vi "create Legend.vi"(8 "error in (no error)":errorcluster, 11 "Chart Options":T1={"ChartName"="Chart", "BorderDashStyle"=enum."Solid", "Bordercolor"=0, "Title"={"Title"="", "TitleFontSize"=0.0, "fontName"="Arial", "font Color"=0, "Docking"=enum."Top"}, "Legend"={"Docking"=enum."None", "BorderDashStyle"=enum."Solid", "BGKcolor"=0, "BGKalpha"=103, "Title"="", "TitleSeparator"=enum."ThickLine"}} {"Legend"."BGKalpha" scale=0.0..255.0; "Title"."TitleFontSize" min=4.0 max=100.0}) -> (0 "error out":errorcluster, 3 ".NET MSChart Legend":refnum<k24>)   [LabVIEW 2015, in "Graph Extensions MSChart.lvlib"]
uses:
  Graph Extensions MSChart.lvlib
  System.Windows.Forms.DataVisualization
  Controls/Chart.ctl
  Controls/Title.ctl
  Controls/Legend.ctl
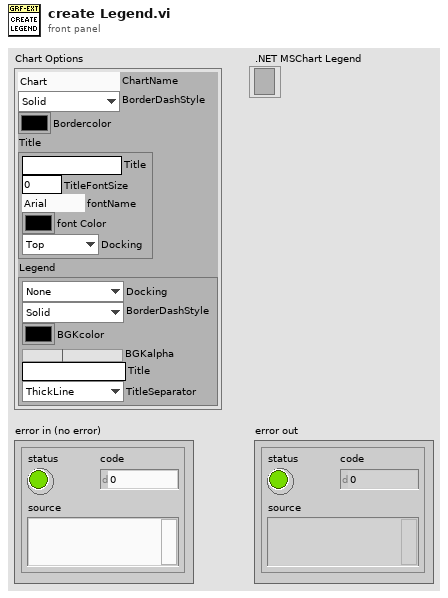
[diagram p1: front panel]
types:
  T1 = typedef "Graph Extensions MSChart.lvlib/Chart.ctl" = cluster{"ChartName":string, "BorderDashStyle":enum16{"NotSet", "Dash", "DashDot", "DashDotDot", "Dot", "Solid"}, "Bordercolor":u32, "Title":T2, "Legend":T3}
  T2 = typedef "Graph Extensions MSChart.lvlib/Title.ctl" = cluster{"Title":string, "TitleFontSize":dbl, "fontName":string, "font Color":u32, "Docking":enum16{"Top", "Right", "Bottom", "Left"}}
  T3 = typedef "Graph Extensions MSChart.lvlib/Legend.ctl" = cluster{"Docking":enum16{"None", "Top", "Right", "Bottom", "Left"}, "BorderDashStyle":enum16{"NotSet", "Dash", "DashDot", "DashDotDot", "Dot", "Solid"}, "BGKcolor":u32, "BGKalpha":u8, "Title":string, "TitleSeparator":enum16{"None", "Line", "ThickLine", "DoubleLine", "DashLine", "DotLine", "GradientLine", "ThickGradientLine"}}
  T4 = enum16{"NotSet", "Dash", "DashDot", "DashDotDot", "Dot", "Solid"}
  T5 = enum16{"None", "Line", "ThickLine", "DoubleLine", "DashLine", "DotLine", "GradientLine", "ThickGradientLine"}
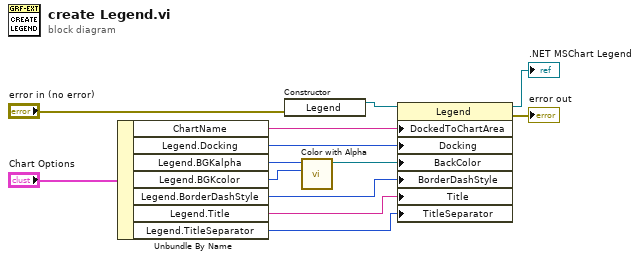
[diagram p0: block diagram]
diagram:
  n1 = Unbundle By Name("Chart Options") -> ("ChartName"=w7:string, "Legend.Docking"=w6:enum16{"None", "Top", "Right", "Bottom", "Left"}, "Legend.BGKalpha"=w4:u8, "Legend.BGKcolor"=w5:u32, "Legend.BorderDashStyle"=w3:T4, "Legend.Title"=w2:string, "Legend.TitleSeparator"=w1:T5)
  n2 = constructor class="Legend"(error in="error in (no error)") -> (reference out=w9:refnum<k24>)  [unwired: 2 in, 2 out]
  n3 = call "Color with Alpha.vi"("Color"=w5, "alpha"=w4) -> (".NET color Refnum out"=w11:refnum<k24>)  [unwired: 9 in]
  n4 = property class="Legend"(reference=w9, "DockedToChartArea"=w7, "Docking"=w6, "BackColor"=w11, "BorderDashStyle"=w3, "Title"=w2, "TitleSeparator"=w1) -> (reference out=→".NET MSChart Legend":refnum<k24>, error out=→"error out":errorcluster)  [unwired: 1 in]
